vi "Get Type.vi"(11 "TimestampPanel in":refnum<class "TimestampPanel.lvclass">) -> (2 "Type":refnum<class "Type.lvclass">)   [LabVIEW 2020, in "Conditum-Tools.lvlib" / "TimestampPanel.lvclass"]
uses:
  TimestampPanel.lvclass
  Conditum-Clone/Columns/Type/Type.lvclass
  TimestampPanel.lvclass/TimestampPanel.ctl
  Conditum-Clone/Columns/Timestamp/Timestamp.lvclass
  C:/dev/lv20CE/lv-conditum-tools/Conditum-Clone/Columns/Type/Type.lvclass
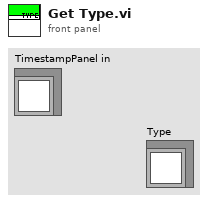
[diagram p1: front panel]
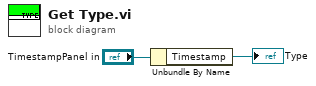
[diagram p0: block diagram]
diagram:
  n1 = Unbundle By Name("TimestampPanel in") -> ("Timestamp"=→"Type":refnum<class "Timestamp.lvclass">)
